vi "Initialize Main Page.vi"(8 "error in (no error)":errorcluster, 10 "Main Page Controls":T2, 11 "Item Ref in":T1 format="%.0x") -> (0 "error out":errorcluster, 3 "Item Ref out":T1 format="%.0x")   [LabVIEW 2017, in "SLSC Switch System Explorer.lvlib"]
uses:
  SLSC Switch System Explorer.lvlib
  Main Page Controls.ctl
  <vilib>/NI Veristand/Custom Device API/Custom Device Item Ref.ctl
  <vilib>/SLSC_Switch/Get Topologies (Simulate).vi
  Scripting/SLSC Switch Scripting.lvlib
  <vilib>/SLSC_Switch/SLSC Switch.lvlib
  <vilib>/NI Veristand/Custom Device API/Custom Device API.lvlib
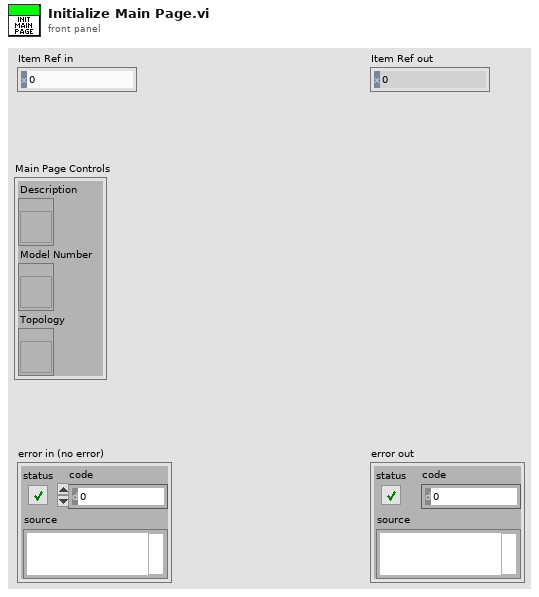
[diagram p1: front panel]
types:
  T1 = typedef "Custom Device API.lvlib/Custom Device Item Ref.ctl" = u64
  T2 = typedef "SLSC Switch System Explorer.lvlib/Main Page Controls.ctl" = cluster{"Description":refnum<vi>, "Model Number":refnum<vi>, "Topology":refnum<vi>}
  T3 = typedef "SLSC Switch Scripting.lvlib/SLSC Switch All Properties.ctl" = cluster{"Model":string, "Resource":string, "Topology":string, "Capabilities":string, "Description":string}
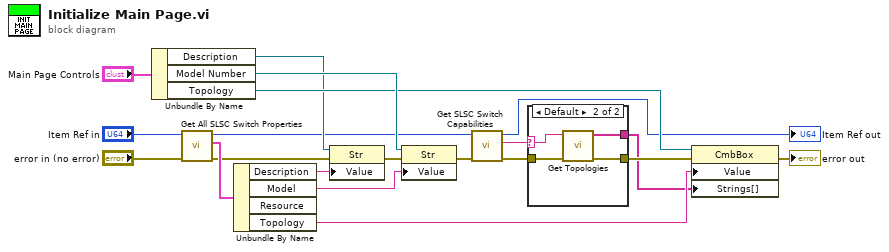
[diagram p0: block diagram]
diagram:
  n1 = Unbundle By Name("Main Page Controls") -> ("Description"=w12:refnum<vi>, "Model Number"=w19:refnum<vi>, "Topology"=w15:refnum<vi>)
  n2 = call "Get All SLSC Switch Properties.vi"("error in (no error)"="error in (no error)", "SLSC Switch Custom Device Ref in"="Item Ref in") -> ("error out"=w8:errorcluster, "SLSC Switch All Properties"=w18:T3, "SLSC Switch Custom Device Ref out"=w5:T1)  [unwired: 7 in]
  n3 = Unbundle By Name(w18) -> ("Description"=w11:string, "Model"=w17:string, "Topology"=w16:string)  [unwired: 1 out]
  n4 = property class="Str"(reference=w12, error in=w8, "Value"=w11) -> (error out=w13:errorcluster)  [unwired: 1 out]
  n5 = property class="Str"(reference=w19, error in=w13, "Value"=w17) -> (error out=w4:errorcluster)  [unwired: 1 out]
  n6 = call "Get SLSC Switch Capabilities.vi"("error in (no error)"=w4, "SLSC Switch Custom Device Ref in"=w5) -> ("error out"=w6:errorcluster, "Capabilities"=w7:string, "SLSC Switch Custom Device Ref out"=→"Item Ref out":T1)  [unwired: 7 in]
  n7 = case shown="Default" w7 {
    selector: w7 -> [_ w25]
    tunnel: w6 -> [w21 w24]
    tunnel: [w21 w23] -> w3
    tunnel: [_ w22] -> w2
    frame "" {
    }
    frame Default {
      n8 = call-poly <vilib>:"Get Topologies.vi"("error in (no error)"=w24, "switches json"=w25) -> ("error out"=w23:errorcluster, "topologies"=w22:string[])  [unwired: 8 in]
    }
  }
  n9 = property class="CmbBox"(reference=w15, error in=w3, "Value"=w16, "Strings[]"=w2) -> (error out=→"error out":errorcluster)  [unwired: 1 out]
